vi "Reject redundant relative timestamps.vi"(9 "Acquisition time unknown":bool, 10 "Experiment Header's Statistics":T1, 11 "Frame relative times array":dbl[](array[numeric])) -> (0 "Difference (points)":i32, 1 "Elements to keep":bool[](array[boolean]), 2 "Number of elements to keep":i32, 3 "Frame relative times array":dbl[](array[numeric]))   [LabVIEW 2020]
uses:
  Typedefs/Test header stats cluster.ctl
  <userlib>/_OpenG.lib/array/array.llb/Conditional Auto-Indexing Tunnel (DBL)__ogtk.vi
panel:
  out "Original number of points":i32
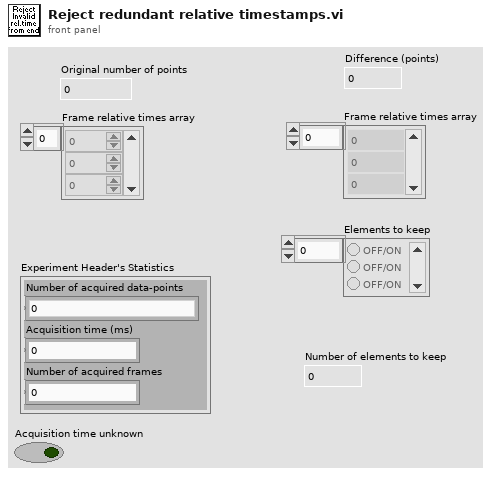
[diagram p1: front panel]
types:
  T1 = typedef "Test header stats cluster.ctl" = cluster{"Number of acquired data-points":dbl, "Acquisition time (ms)":dbl, "Number of acquired frames":dbl}
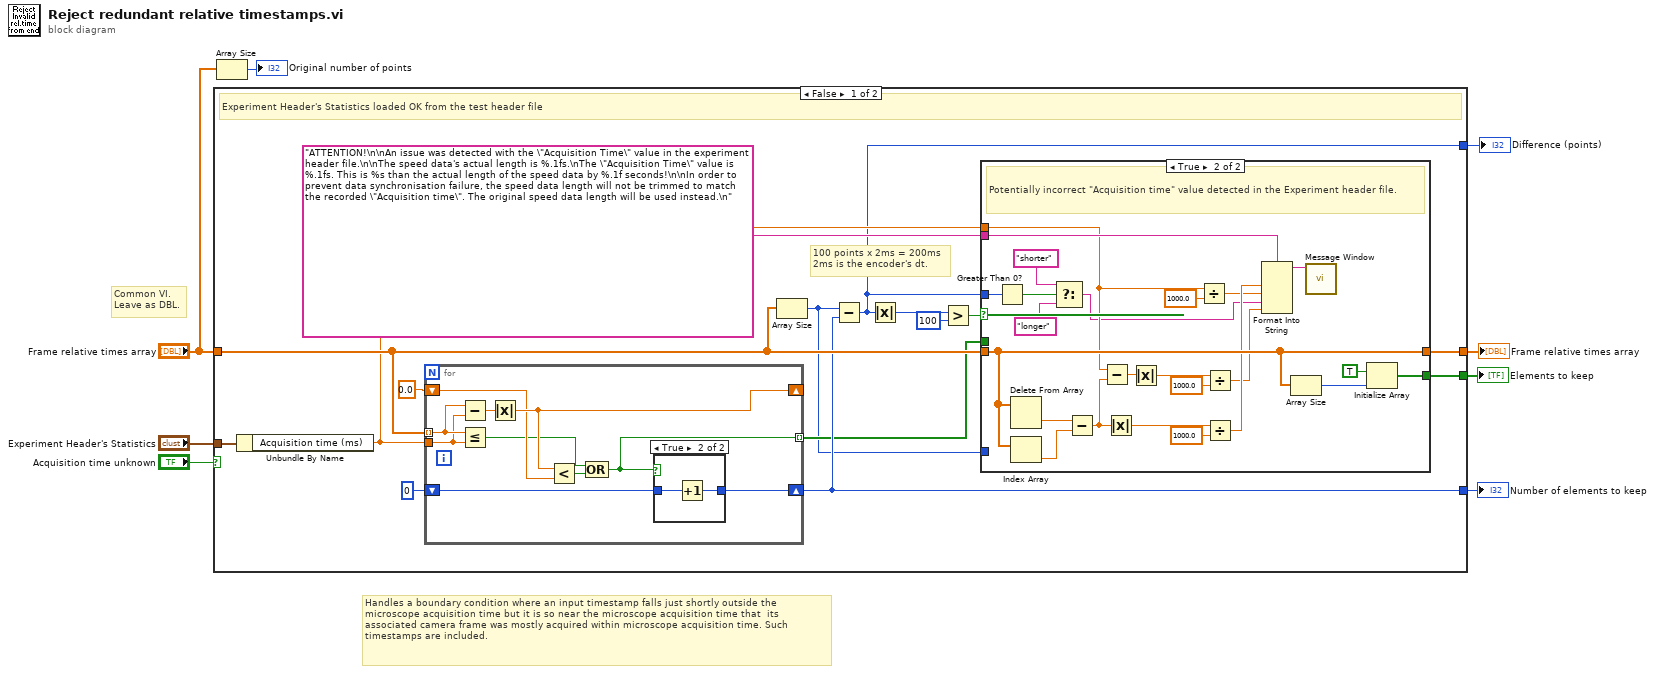
[diagram p0: block diagram]
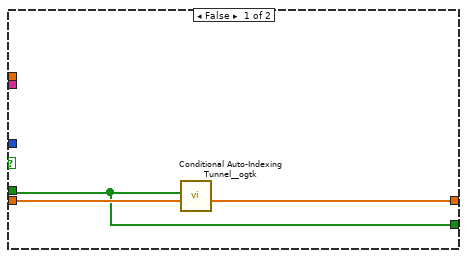
[diagram p2: hidden frame]
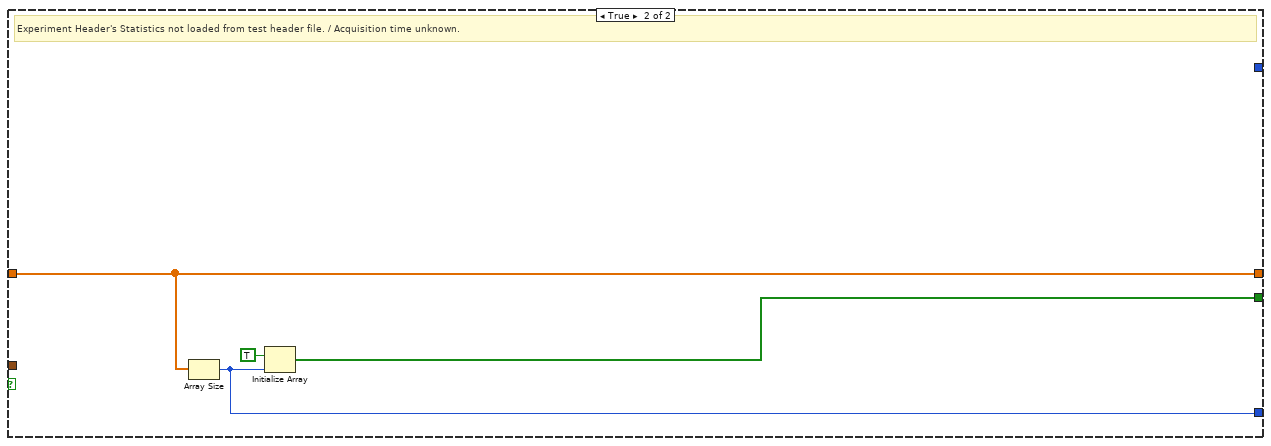
[diagram p4: hidden frame]
diagram:
  # "Handles a boundary condition where an input timestamp falls just shortly outside the microscope acquisition time but it is so near the microscope acquisition time that  its associated camera frame was mostly acquired within microscope acquisition time. Such timestamps are included."
  # "Common VI.\nLeave as DBL."
  n1 = case shown="False" "Acquisition time unknown" {
    tunnel: "Experiment Header's Statistics" -> [w23 _]
    tunnel: "Frame relative times array" -> [w19 w67]
    tunnel: [w22 w67] -> w7
    tunnel: [w12 w65] -> w6
    tunnel: [w17 w64] -> w4
    tunnel: [w9 _] -> w1
    frame False {
      # "100 points x 2ms = 200ms\n2ms is the encoder's dt."
      # "Experiment Header's Statistics loaded OK from the test header file"
      n2 = Unbundle By Name(w23) -> ("Acquisition time (ms)"=w11:dbl)
      n3 = for {
        tunnel: w19 -> [w58] mode=indexing
        tunnel: w11 -> [w57]
        tunnel: [w51] -> w13 mode=indexing
        shift-right: [w59] -> w17
        shift-left: 0 -> [w60]
        shift-right: [w55] -> _
        shift-left: 0.0 -> [w54]
        n4 = Subtract(x=w58, y=w57) -> (x-y=w56:dbl)
        n5 = Less Or Equal?(x=w58, y=w57) -> (x <= y?=w52:bool)
        n6 = Absolute Value(x=w56) -> (abs(x)=w55:dbl)
        n7 = Less?(x=w55, y=w54) -> (x < y?=w53:bool)
        n8 = Compound Arithmetic op=OR(w52, w53) -> (w51:bool)
        n9 = case shown="True" w51 {
          tunnel: w60 -> [w61 w63]
          tunnel: [w61 w62] -> w59
          frame False {
          }
          frame True {
            n10 = Increment(x=w63) -> (x+1=w62:i32)
          }
        }
      }
      n11 = Array Size(array=w19) -> (size(s)=w10:i32)
      n12 = Subtract(x=w10, y=w17) -> (x-y=w9:i32)
      n13 = Absolute Value(x=w9) -> (abs(x)=w14:i32)
      n14 = Greater?(x=w14, y=100) -> (0:w16:bool)
      n15 = case shown="True" w16 {
        tunnel: [w26 w38] -> w22
        tunnel: w13 -> [w24 _]
        tunnel: w19 -> [w25 w38]
        tunnel: w9 -> [_ w50]
        tunnel: "ATTENTION!\n\nAn issue was detected with the \"Acquisition Time\" value in the experiment header file.\n\nThe speed data's actual length is %.1fs.\nThe \"Acquisition Time\" value is %.1fs. This is %s than the actual length of the speed data by %.1f seconds!\n\nIn order to prevent data synchronisation failure, the speed data length will not be trimmed to match the recorded \"Acquisition time\". The original speed data length will be used instead.\n" ("Message string") -> [_ w49]
        tunnel: [w24 w41] -> w12
        tunnel: w11 -> [_ w35]
        tunnel: w10 -> [_ _]
        frame False {
          n16 = call-poly <userlib>:"Conditional Auto-Indexing Tunnel__ogtk.vi"("Array in"=w25, "Elements to keep"=w24) -> ("Filtered Array out"=w26:dbl[])  [unwired: 5 in]
        }
        frame True {
          # "Potentially incorrect \"Acquisition time\" value detected in the Experiment header file."
          n17 = Greater Than 0?(x=w50) -> (x > 0?=w48:bool)
          n18 = Delete From Array(array=w38) -> (deleted portion=w37:dbl)  [unwired: 2 in, 1 out]
          n19 = Index Array(array=w38) -> (element=w36:dbl)  [unwired: 1 in]
          n20 = Select(t="shorter" ("Message string"), s=w48, f="longer") -> (s? t:f=w28:string)
          n21 = Subtract(x=w37, y=w36) -> (x-y=w32:dbl)
          n22 = Subtract(x=w35, y=w32) -> (x-y=w34:dbl)
          n23 = Absolute Value(x=w32) -> (abs(x)=w31:dbl)
          n24 = Absolute Value(x=w34) -> (abs(x)=w33:dbl)
          n25 = Divide(x=w35, y=1000.0) -> (x/y=w29:dbl)
          n26 = Divide(x=w33, y=1000.0) -> (x/y=w27:dbl)
          n27 = Divide(x=w31, y=1000.0) -> (x/y=w30:dbl)
          n28 = Format Into String(format string=w49, w30, w29, w28, w27) -> (resulting string=w45:string)  [unwired: 2 in, 1 out]
          n29 = Array Size(array=w38) -> (size(s)=w42:i32)
          n30 = call "Message Window.vi"("Message string"=w45) -> ()  [unwired: 10 in, 1 out]
          n31 = Initialize Array(TRUE ("No test header file"), w42) -> (w41:bool[])
        }
      }
    }
    frame True {
      # "Experiment Header's Statistics not loaded from test header file. / Acquisition time unknown."
      n32 = Array Size(array=w67) -> (size(s)=w64:i32)
      n33 = Initialize Array(TRUE ("No test header file"), w64) -> (w65:bool[])
    }
  }
  "Frame relative times array" <- w7
  "Elements to keep" <- w6
  "Number of elements to keep" <- w4
  "Difference (points)" <- w1
  n34 = Array Size(array="Frame relative times array") -> (size(s)=→"Original number of points":i32)
